vi "Recipe_To_Display.vi"(0 "Recipes":string[][](array[string])=[["1", "Rice", "66PL10", "12PL3", "10PL4"], ["2", "Frozen Dinner", "5PL8", "10PL2", ""], ["3", "Popcorn", "5PL3", "", ""]], 1 "State In":T1=enum."Idle", 5 "Recipe":i32, 7 "Step In":i32, 9 "Elaspsed Time":dbl, 11 "error in (no error)":errorcluster) -> (3 "State Out":T1, 4 "Display Out":string, 8 "Step Out":i32, 10 "Elaspsed Time":dbl, 15 "error out":errorcluster)   [LabVIEW 2026]
uses:
  controls/State_Enum.ctl
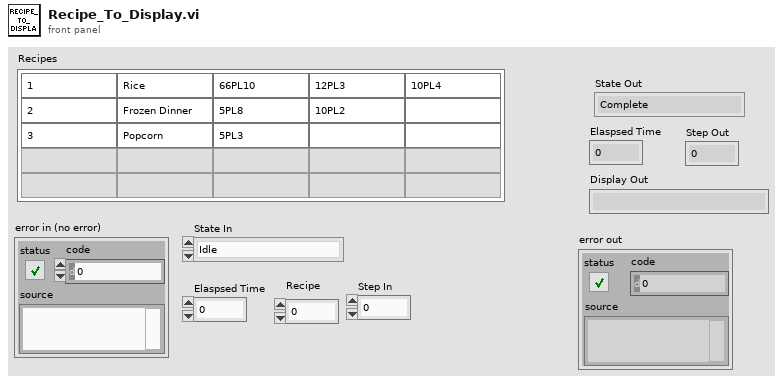
[diagram p1: front panel]
types:
  T1 = typedef "State_Enum.ctl" = enum16{"Complete", "Run", "Idle"}
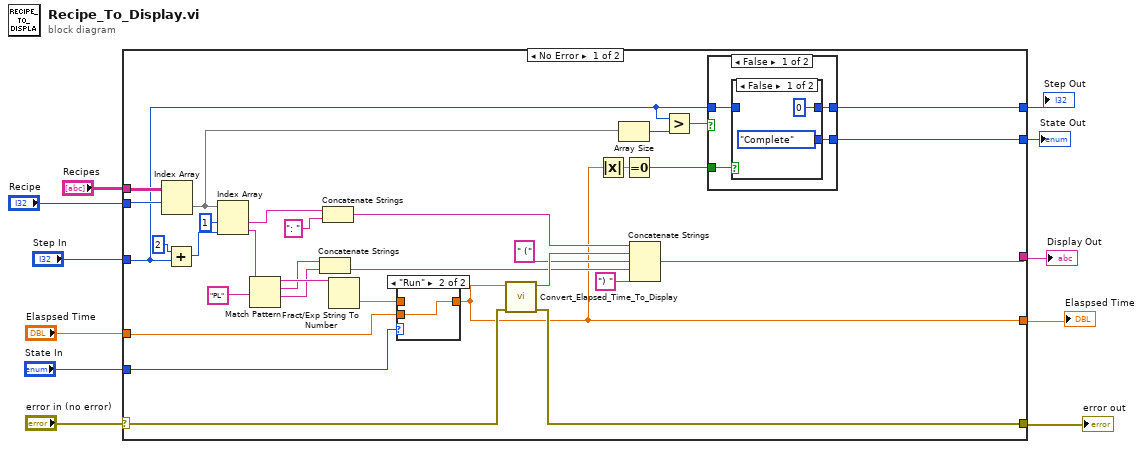
[diagram p0: block diagram]
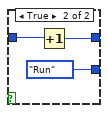
[diagram p2: hidden frame]
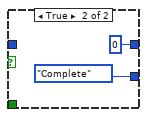
[diagram p3: hidden frame]
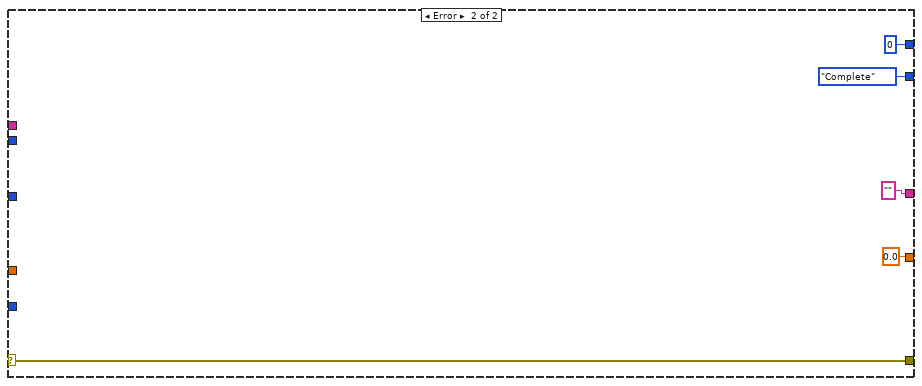
[diagram p5: hidden frame]
diagram:
  n1 = case shown="No Error" "error in (no error)" {
    selector: "error in (no error)" -> [w22 w61]
    tunnel: "Recipes" -> [w43 _]
    tunnel: [w21 w61] -> w10
    tunnel: [w31 ""] -> w9
    tunnel: "Step In" -> [w12 _]
    tunnel: "Recipe" -> [w27 _]
    tunnel: [w17 0.0] -> w5
    tunnel: "Elaspsed Time" -> [w23 _]
    tunnel: "State In" -> [w25 _]
    tunnel: [w14 0] -> w1
    tunnel: [w13 State_Enum."Complete" ("State")] -> w2
    frame No Error {
      n2 = Index Array(array=w43, index (row)=w27) -> (element=w19:string[])  [unwired: 1 in]
      n3 = Add(x=2, y=w12) -> (x+y=w29:i32)
      n4 = Index Array(array=w19, index #1=1 ("index"), index #2=w29) -> (element #1=w40:string, element #2=w30:string)
      n5 = Match Pattern(string=w30, regular expression="PL") -> (before substring=w39:string, match substring=w35:string, after substring=w34:string)  [unwired: 1 in, 1 out]
      n6 = Concatenate Strings(w35, w34) -> (w33:string)
      n7 = Concatenate Strings(w40, ": ") -> (w38:string)
      n8 = Fract/Exp String To Number(string=w39) -> (number=w24:dbl)  [unwired: 3 in, 1 out]
      n9 = case shown="\"Run\"" w25 {
        tunnel: w24 -> [w55 _]
        tunnel: [w55 w56] -> w17
        tunnel: w23 -> [_ w56]
        frame "Idle", Default {
        }
        frame "Run" {
        }
      }
      n10 = call "Convert_Elapsed_Time_To_Display.vi"("error in (no error)"=w22, "Elapsed Time"=w17) -> ("error out"=w21:errorcluster, "Display Out"=w37:string)  [unwired: 8 in]
      n11 = Absolute Value(x=w17) -> (abs(x)=w20:dbl)
      n12 = Array Size(array=w19) -> (size(s)=w18:i32)
      n13 = Equal To 0?(x=w20) -> (x = 0?=w15:bool)
      n14 = Concatenate Strings(w38, w37, " (", w33, ") ") -> (w31:string)
      n15 = Greater?(x=w12, y=w18) -> (0:w16:bool)
      n16 = case shown="False" w16 {
        tunnel: w15 -> [w47 _]
        tunnel: w12 -> [w46 _]
        tunnel: [w45 0] -> w14
        tunnel: [w44 State_Enum."Complete" ("State")] -> w13
        frame False {
          n17 = case shown="False" w47 {
            tunnel: [0 w50] -> w45
            tunnel: w46 -> [_ w51]
            tunnel: [State_Enum."Complete" ("State") State_Enum."Run" ("State")] -> w44
            frame False {
            }
            frame True {
              n18 = Increment(x=w51) -> (x+1=w50:i32)
            }
          }
        }
        frame True {
        }
      }
    }
    frame Error {
    }
  }
  "error out" <- w10
  "Display Out" <- w9
  "Elaspsed Time" <- w5
  "State Out" <- w2
  "Step Out" <- w1
